vi "Anritsu VNA Config Test.vi"(4 "error in (no error)":errorcluster, 6 "Configuration":T1={"BusType"=enum."GPIB", "GPIB Bus"=0, "GPIB Address"=16, "IP"=0, "COM"=1, "Baud Rate"=enum."9600", "USB Device"=0, "Instrument S\\N"="", "SCIL Address"=16} {"USB Device" max=31 step=1}, 7 "Str Refnum":refnum<vi>) -> (0 "error out":errorcluster, 3 "Serial Number":string)   [LabVIEW 2011]
uses:
  VNA Configuration.ctl
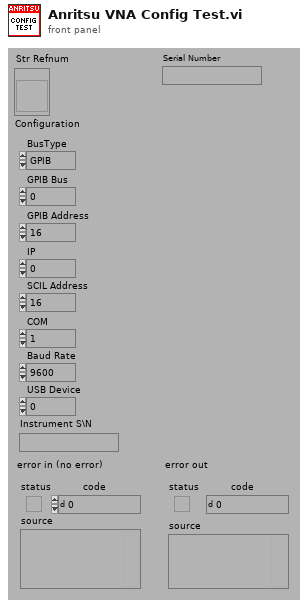
[diagram p1: front panel]
types:
  T1 = typedef "VNA Configuration.ctl" = cluster{"BusType":enum32{"GPIB", "LAN/IP", "Serial", "USB"}, "GPIB Bus":i32, "GPIB Address":i32, "IP":u32, "COM":i32, "Baud Rate":enum32{"300", "600", "1200", "2400", "4800", "9600"}, "USB Device":u32, "Instrument S\\N":string, "SCIL Address":i32}
  T2 = enum32{"300", "600", "1200", "2400", "4800", "9600"}
  T3 = typedef "Anritsu VNA Instrument Info.ctl" = cluster{"Model":string, "Serial":string, "Firmware":string, "Learn String":string}
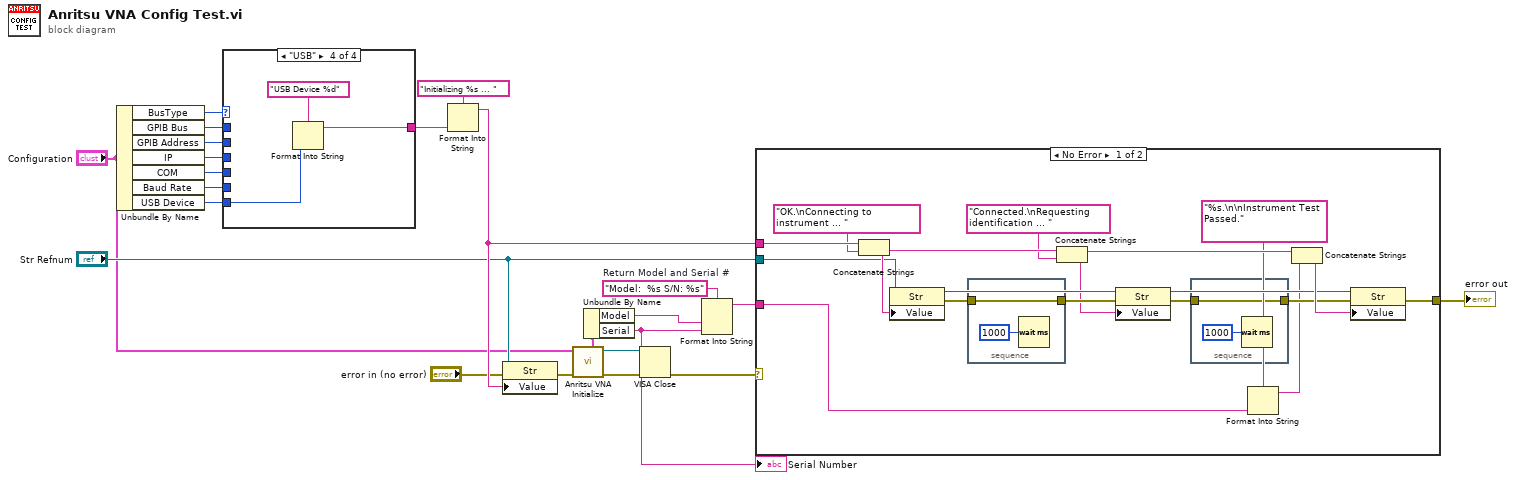
[diagram p0: block diagram]
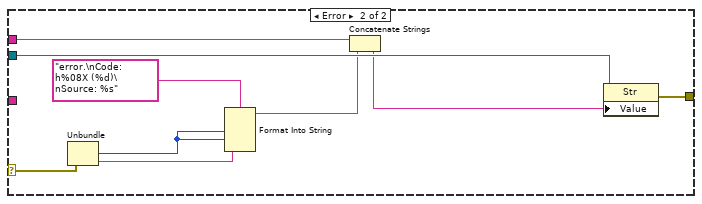
[diagram p2: hidden frame]
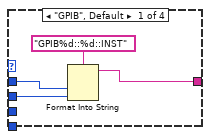
[diagram p3: hidden frame]
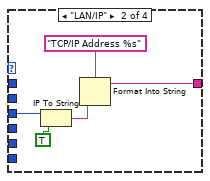
[diagram p4: hidden frame]
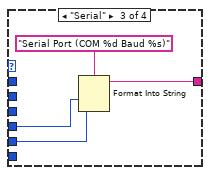
[diagram p5: hidden frame]
diagram:
  w10 = "Model:  %s S/N: %s"  # Return Model and Serial #
  n1 = Unbundle By Name("Configuration") -> ("BusType"=w22:enum32{"GPIB", "LAN/IP", "Serial", "USB"}, "GPIB Bus"=w21:i32, "GPIB Address"=w20:i32, "IP"=w19:u32, "COM"=w18:i32, "Baud Rate"=w3:T2, "USB Device"=w2:u32)
  n2 = case shown="\"USB\"" w22 {
    tunnel: w21 -> [w26 _ _ _]
    tunnel: w20 -> [w25 _ _ _]
    tunnel: w19 -> [_ w31 _ _]
    tunnel: w18 -> [_ _ w35 _]
    tunnel: [w24 w28 w34 w38] -> w17
    tunnel: w3 -> [_ _ w33 _]
    tunnel: w2 -> [_ _ _ w37]
    frame "GPIB", Default {
      n3 = Format Into String(format string="GPIB%d::%d::INST", w26, w25) -> (resulting string=w24:string)  [unwired: 2 in, 1 out]
    }
    frame "LAN/IP" {
      n4 = IP To String(1:TRUE, 2:w31) -> (0:w30:string)
      n5 = Format Into String(format string="TCP/IP Address %s", w30) -> (resulting string=w28:string)  [unwired: 2 in, 1 out]
    }
    frame "Serial" {
      n6 = Format Into String(format string="Serial Port (COM %d Baud %s)", w35, w33) -> (resulting string=w34:string)  [unwired: 2 in, 1 out]
    }
    frame "USB" {
      n7 = Format Into String(format string="USB Device %d", w37) -> (resulting string=w38:string)  [unwired: 2 in, 1 out]
    }
  }
  n8 = Format Into String(format string="Initializing %s ... ", w17) -> (resulting string=w16:string)  [unwired: 2 in, 1 out]
  n9 = property class="Str"(reference="Str Refnum", error in="error in (no error)", "Value"=w16) -> (error out=w12:errorcluster)  [unwired: 1 out]
  n10 = call "Anritsu VNA Initialize.vi"("error in (no error)"=w12, "Configuration"="Configuration") -> ("error out"=w8:errorcluster, "dup VISA Resource Name"=w6:refnum<visa-resource-name>, "Anritsu VNA"=w5:T3)  [unwired: 7 out]
  n11 = Unbundle By Name(w5) -> ("Model"=w9:string, "Serial"=w1:string)
  "Serial Number" <- w1
  n12 = VISA Close(VISA resource name=w6, error in (no error)=w8) -> (error out=w7:errorcluster)
  n13 = Format Into String(format string=w10, w9, w1) -> (resulting string=w4:string)  [unwired: 2 in, 1 out]
  n14 = case shown="No Error" w7 {
    selector: w7 -> [_ w66]
    tunnel: w16 -> [w52 w69]
    tunnel: [w45 w68] -> w15
    tunnel: "Str Refnum" -> [w43 w65]
    tunnel: w4 -> [w40 _]
    frame No Error {
      n15 = Concatenate Strings(w52, "OK.\nConnecting to instrument ... ") -> (w50:string)
      n16 = property class="Str"(reference=w43, "Value"=w50) -> (reference out=w54:refnum<vi>, error out=w56:errorcluster)  [unwired: 1 in]
      n17 = stacked-sequence {
        tunnel: w56 -> [w59]
        tunnel: [w59] -> w55
        frame #0 {
          n18 = Wait (ms)(milliseconds to wait=u32 1000) -> ()  [unwired: 1 out]
        }
      }
      n19 = Concatenate Strings(w50, "Connected.\nRequesting identification ... ") -> (w46:string)
      n20 = property class="Str"(reference=w54, error in=w55, "Value"=w46) -> (reference out=w44:refnum<vi>, error out=w53:errorcluster)
      n21 = stacked-sequence {
        tunnel: w53 -> [w57]
        tunnel: [w57] -> w47
        frame #0 {
          n22 = Wait (ms)(milliseconds to wait=u32 1000) -> ()  [unwired: 1 out]
        }
      }
      n23 = Format Into String(format string="%s.\n\nInstrument Test Passed.", w40) -> (resulting string=w41:string)  [unwired: 2 in, 1 out]
      n24 = Concatenate Strings(w46, w41) -> (w48:string)
      n25 = property class="Str"(reference=w44, error in=w47, "Value"=w48) -> (error out=w45:errorcluster)  [unwired: 1 out]
    }
    frame Error {
      n26 = Unbundle(w66) -> ("code"=w64:i32, "source"=w63:string)  [unwired: 1 out]
      n27 = Format Into String(format string="error.\nCode:  h%08X (%d)\nSource: %s", w64, w64, w63) -> (resulting string=w62:string)  [unwired: 2 in, 1 out]
      n28 = Concatenate Strings(w69, w62) -> (w61:string)
      n29 = property class="Str"(reference=w65, "Value"=w61) -> (error out=w68:errorcluster)  [unwired: 1 in, 1 out]
    }
  }
  "error out" <- w15
